vi "AlliGator Get Phasor Ratio Interpolated Color Scale.vi"(8 "Error In":errorcluster, 9 "Reference 2 Color":u32, 11 "Reference 1 Color":u32) -> (0 "Error Out":errorcluster, 3 "Interpolated Color Scale Definition":T1)   [LabVIEW 2021, in "AlliGator Settings.lvlib"]
doc: "Builds a <B>Interpolated Color Scale Definition</B> based on the colors associated with both references."
uses:
  AlliGator Settings.lvlib
  Palette/Interpolated Color Scale Definition.ctl
  Palette/Palette.lvlib
panel:
  # "see the AlliGator License on the block diagram (Ctrl+E or Window:Show Block Diagram)"
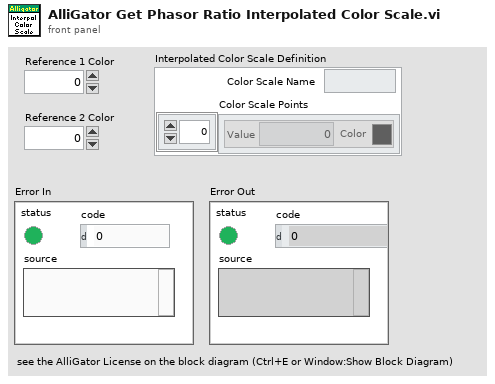
[diagram p1: front panel]
types:
  T1 = typedef "Palette.lvlib/Interpolated Color Scale Definition.ctl" = cluster{"Color Scale Points":cluster{"Value":dbl, "Color":u32}[], "Color Scale Name":string}
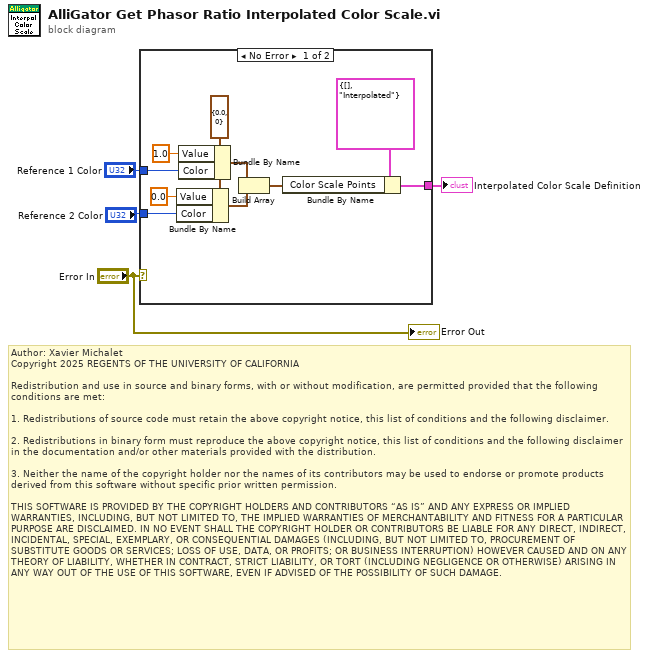
[diagram p0: block diagram]
diagram:
  # "Author: Xavier Michalet\nCopyright 2025 REGENTS OF THE UNIVERSITY OF CALIFORNIA\n\nRedistribution and use in source and binary forms, with or without modification, are permitted provided that the following conditions are met:\n\n1. Redistributions of source code must retain the above copyright notice, this list of conditions and the following disclaimer.\n\n2. Redistributions in binary form must reproduce the above copyright notice, this list of conditions and the following disclaimer in the documentation and/or other materials provided with the distribution.\n\n3. Neither the name of the copyright holder nor the names of its contributors may be used to endorse or promote products derived from this software without specific prior written permission.\n\nTHIS SOFTWARE IS PROVIDED BY THE COPYRIGHT HOLDERS AND CONTRIBUTORS “AS IS” AND ANY EXPRESS OR IMPLIED WARRANTIES, INCLUDING, BUT NOT LIMITED TO, THE IMPLIED WARRANTIES OF MERCHANTABILITY AND FITNESS FOR A PARTICULAR PURPOSE ARE DISCLAIMED. IN NO EVENT SHALL THE COPYRIGHT HOLDER OR CONTRIBUTORS BE LIABLE FOR ANY DIRECT, INDIRECT, INCIDENTAL, SPECIAL, EXEMPLARY, OR CONSEQUENTIAL DAMAGES (INCLUDING, BUT NOT LIMITED TO, PROCUREMENT OF SUBSTITUTE GOODS OR SERVICES; LOSS OF USE, DATA, OR PROFITS; OR BUSINESS INTERRUPTION) HOWEVER CAUSED AND ON ANY THEORY OF LIABILITY, WHETHER IN CONTRACT, STRICT LIABILITY, OR TORT (INCLUDING NEGLIGENCE OR OTHERWISE) ARISING IN ANY WAY OUT OF THE USE OF THIS SOFTWARE, EVEN IF ADVISED OF THE POSSIBILITY OF SUCH DAMAGE."
  n1 = case shown="No Error" "Error In" {
    tunnel: "Reference 1 Color" -> [w12 _]
    tunnel: "Reference 2 Color" -> [w10 _]
    tunnel: [w5 _] -> w1
    frame No Error {
      w8 = cluster{"Value":dbl, "Color":u32} {"Value"=0.0, "Color"=0} ("Color Scale Point")
      n2 = Bundle By Name(cluster=w8, "Value"=0.0, "Color"=w10) -> (w7:cluster{"Value":dbl, "Color":u32})
      n3 = Bundle By Name(cluster=w8, "Value"=1.0, "Color"=w12) -> (w9:cluster{"Value":dbl, "Color":u32})
      n4 = Build Array(w9, w7) -> (w6:cluster{"Value":dbl, "Color":u32}[])
      n5 = Bundle By Name(cluster=T1 {"Color Scale Points"=[], "Color Scale Name"="Interpolated"} ("Interpolated Color Scale Definition"), "Color Scale Points"=w6) -> (w5:T1)
    }
    frame Error {
    }
  }
  "Interpolated Color Scale Definition" <- w1
  "Error Out" <- "Error In"
